vi "InsetRect.vi"(1 "dv":i16=1, 2 "dh":i16=1, 3 "rect":T1) -> (0 "inset rect":T1)   [LabVIEW 2020]
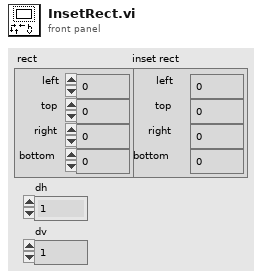
[diagram p1: front panel]
types:
  T1 = cluster{"left":i16, "top":i16, "right":i16, "bottom":i16}
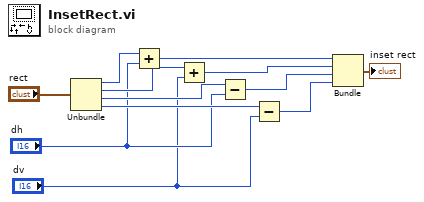
[diagram p0: block diagram]
diagram:
  n1 = Unbundle("rect") -> ("left"=w10:i16, "top"=w8:i16, "right"=w6:i16, "bottom"=w4:i16)
  n2 = Add(x=w10, y="dh") -> (x+y=w9:i16)
  n3 = Add(x=w8, y="dv") -> (x+y=w7:i16)
  n4 = Subtract(x=w6, y="dh") -> (x-y=w5:i16)
  n5 = Subtract(x=w4, y="dv") -> (x-y=w3:i16)
  n6 = Bundle(w9, w7, w5, w3) -> (→"inset rect":cluster{i16, i16, i16, i16})  [unwired: 1 in]
